vi "General Error Handler Core CORE__Copy.vi"(0 "[error code] (0)":i32 format="%0.0f", 1 "[error source] (\" \")":string, 3 "String to Format (not a refnum)":refnum<vi>, 4 "type of dialog (OK msg:1)":T2=enum."OK message", 5 "error in (no error)":errorcluster, 6 "[user-defined codes]":i32[](array[numeric]), 7 "[exception action] (none:0)":i32(ring) items=["no exception", "cancel error on match", "set error on match"], 8 "ni.com link visible (F)":bool, 9 "prompts":T1={"Error %d occurred at %s"="Error %d occurred at %s", "Warning %d occurred at %s"="Warning %d occurred at %s", "Possible reasons: %s"="<b>Possible reason(s):</b>\\n%s", "Error not listed"="This error code is undefined. Undefined errors might occur for a number of reasons. For example, no one has provided a description for the code, or you might have wired a number that is not an error code to the error code input. \n\nAdditionally, undefined error codes might occur because the error relates to a third-party object, such as the operating system or ActiveX. For these third-party errors, you might be able to obtain a description of the error by searching the Web for the error code (%s) or for its hexadecimal representation (0x%s).", "GetCommError x%lx"="Windows GetCommError:  The hex value of this code is <B>x%04lx</B>.\n\nInterpret it bit-wise as follows:\n<B>x4000</B>: serial port VI error\n<B>x0001</B>: receiving queue overflowed or character was received after end-of-file character\n<B>x0002</B>: character was lost by overwrite\n<B>x0004</B>: parity error\n<B>x0008</B>: framing error\n<B>x0010</B>: break condition\n<B>x0020</B>: CTS timeout\n<B>x0040</B>: DSR timeout\n<B>x0080</B>: RLSD timeout\n<B>x0100</B>: transmission queue was full when new character arrived\n<B>x0200</B>: parallel device timeout\n<B>x0400</B>: parallel device I/O error\n<B>x0800</B>: parallel device not selected\n<B>x1000</B>: parallel device out of paper\n<B>x8000</B>: requested mode is  not supported or the idComDev parameter is invalid.", "Continue"="Continue", "Stop"="Stop", "an unidentified location"="an unidentified location", "No Error"="No Error", "Help"="Why not found?"}, 10 "[user-defined descriptions]":string[](array[string]), 11 "[exception code]":i32 format="%0.0f", 13 "[exception source]":string) -> (12 "stop event propagated":bool, 14 "error?":bool, 15 "code out":i32 format="%0.0f", 17 "source out":string, 18 "message":string=" INSTRUCTIONS:\r\rNormal Use:  When using subVIs that incorporate the error in/error out (or error I/O) structure, place this handler where you want to inform the user of an error, typically at the end of the I/O data path, as the last action of the program.  If the error in error? is ERROR, the handler creates a message describing the error and its source.  If the type of dialog = 1 (default), the message is displayed to the user, who can only acknowledge it.  If the type = 2, the user can acknowledge the message or abort execution; aborting a program with active I/O is not recommended.  If the type = 0, no message is displayed; this is used to process the error programmatically, and the error out cluster elements are wired to individual terminals for that reason.  \r\rOther Use:\n\r\nlocal testing.  To test the error code of a subVI or function that does not have the error I/O structure, you can wire its error code and a source string to the local error code and error source inputs.  If error in error? indicates no error and error code is not equal to 0, the local code and source are substituted for the error in values, and error? is set TRUE (ERROR).", 19 "error out":errorcluster)   [LabVIEW 2020, in "Explain Error Improved Dialog.lvlib"]
uses:
  Explain Error Improved Dialog/Explain Error Improved Dialog.lvlib
  <vilib>/Utility/error.llb/DialogTypeEnum.ctl
  <vilib>/Utility/error.llb/whitespace.ctl
panel:
  # "reinitialize to default to display instructions"
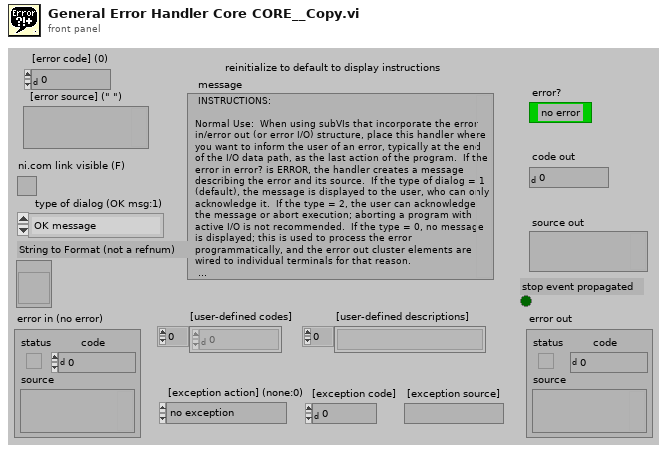
[diagram p1: front panel]
types:
  T1 = cluster{"Error %d occurred at %s":string, "Warning %d occurred at %s":string, "Possible reasons: %s":string, "Error not listed":string, "GetCommError x%lx":string, "Continue":string, "Stop":string, "an unidentified location":string, "No Error":string, "Help":string}
  T2 = typedef "DialogTypeEnum.ctl" = enum16{"no dialog", "OK message", "continue or stop message", "auto error handling dialog", "OK message + warnings", "continue/stop + warnings"}
  T3 = typedef "whitespace.ctl" = u16
  T4 = typedef "TagReturnType.ctl" = enum16{"No Tag", "<err>", "<append>"}
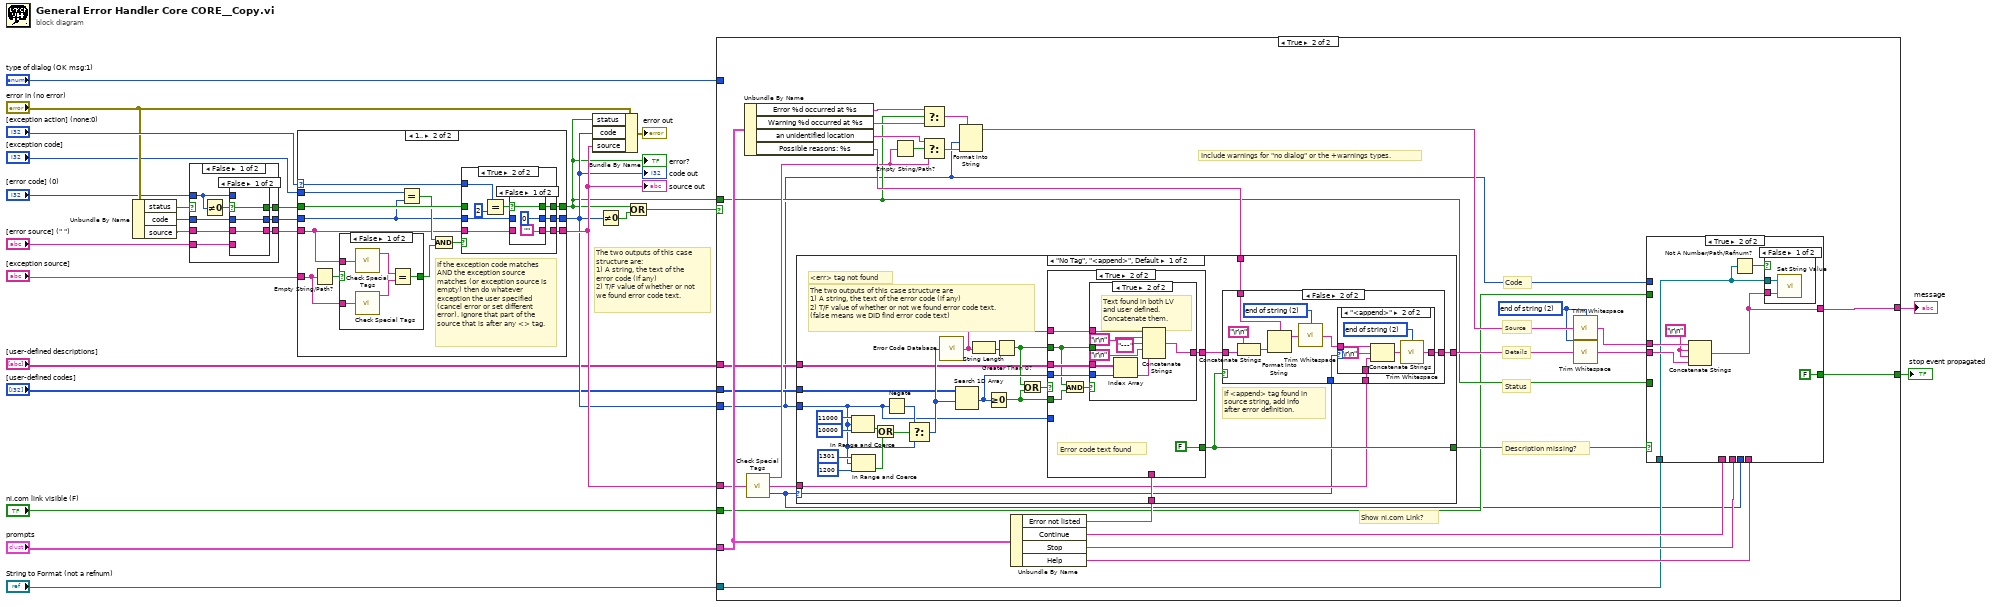
[diagram p0: block diagram]
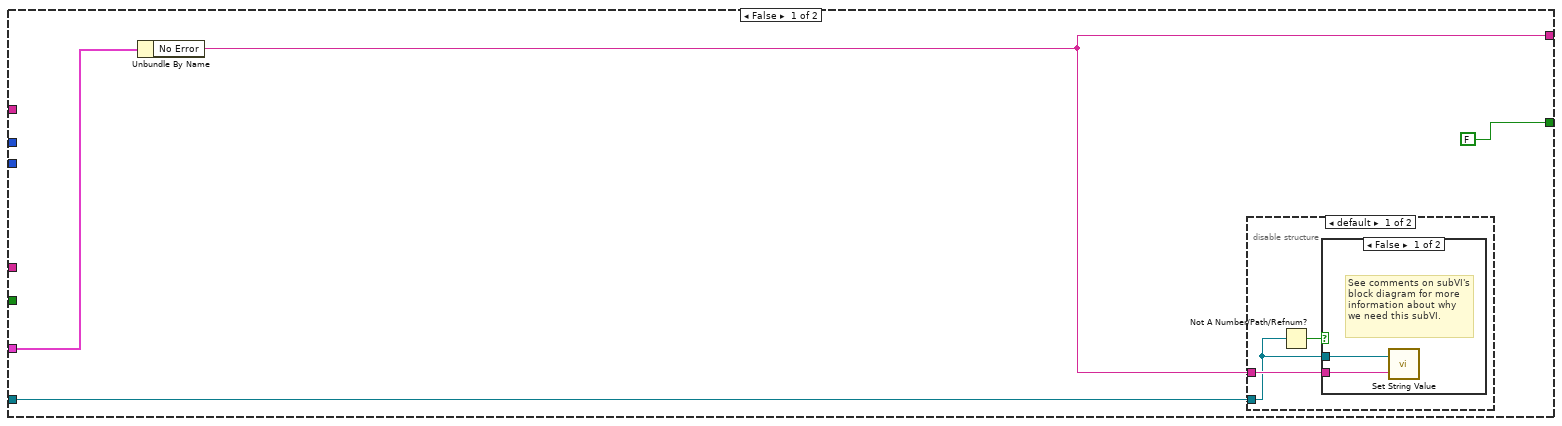
[diagram p8: hidden frame]
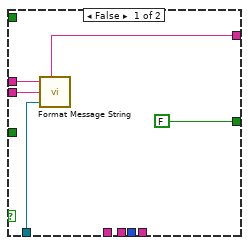
[diagram p11: hidden frame]
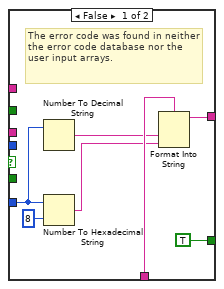
[diagram p15: hidden frame]
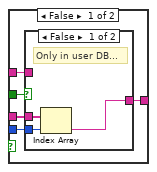
[diagram p16: hidden frame]
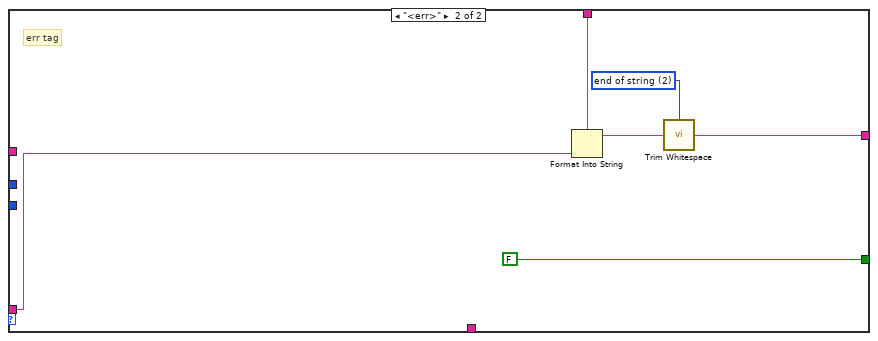
[diagram p18: hidden frame]
diagram:
  # "The two outputs of this case structure are:\n1) A string, the text of the error code (if any)\n2) T/F value of whether or not we found error code text."
  n1 = Unbundle By Name("error in (no error)") -> ("status"=w7:bool, "code"=w21:i32, "source"=w25:string)
  n2 = case shown="False" w7 {
    selector: w7 -> [_ w43]
    tunnel: [w32 w42] -> w23
    tunnel: [w33 w43] -> w22
    tunnel: w21 -> [w29 w42]
    tunnel: [w31 w41] -> w24
    tunnel: w25 -> [w30 w41]
    tunnel: "[error code] (0)" -> [w28 _]
    tunnel: "[error source] (\" \")" -> [w27 _]
    frame False {
      n3 = Not Equal To 0?(x=w28) -> (x != 0?=w34:bool)
      n4 = case shown="False" w34 {
        selector: w34 -> [w37 w40]
        tunnel: [w37 w40] -> w33
        tunnel: w28 -> [_ w39]
        tunnel: [w35 w39] -> w32
        tunnel: w27 -> [_ w38]
        tunnel: [w36 w38] -> w31
        tunnel: w30 -> [w36 _]
        tunnel: w29 -> [w35 _]
        frame False {
        }
        frame True {
        }
      }
    }
    frame True {
    }
  }
  n5 = case shown="1.." "[exception action] (none:0)" {
    selector: "[exception action] (none:0)" -> [_ w51]
    tunnel: [w46 w59] -> w3
    tunnel: w22 -> [w46 w57]
    tunnel: [w45 w58] -> w8
    tunnel: w23 -> [w45 w55]
    tunnel: [w44 w53] -> w18
    tunnel: w24 -> [w44 w49]
    tunnel: "[exception code]" -> [_ w52]
    tunnel: "[exception source]" -> [_ w48]
    frame ..0 {
    }
    frame 1.. {
      # "If the exception code matches AND the exception source matches (or exception source is empty) then do whatever exception the user specified (cancel error or set different error). Ignore that part of the source that is after any <> tag."
      n6 = Empty String/Path?(string/path=w48) -> (empty?=w50:bool)
      n7 = case shown="False" w50 {
        selector: w50 -> [_ w65]
        tunnel: w49 -> [w64 _]
        tunnel: w48 -> [w63 _]
        tunnel: [w62 w65] -> w47
        frame False {
          n8 = call <vilib>:"Check Special Tags.vi"("source"=w64) -> ("Before Tag (source)"=w61:string)  [unwired: 2 out]
          n9 = call <vilib>:"Check Special Tags.vi"("source"=w63) -> ("Before Tag (source)"=w60:string)  [unwired: 2 out]
          n10 = Equal?(x=w61, y=w60) -> (x = y?=w62:bool)
        }
        frame True {
          # "Empty string always matches."
        }
      }
      n11 = Equal?(x=w52, y=w55) -> (x = y?=w56:bool)
      n12 = And(x=w56, y=w47) -> (x .and. y?=w54:bool)
      n13 = case shown="True" w54 {
        tunnel: [w68 w69] -> w59
        tunnel: [w67 w73] -> w58
        tunnel: w57 -> [w68 _]
        tunnel: w55 -> [w67 w72]
        tunnel: w51 -> [_ w76]
        tunnel: [w66 w71] -> w53
        tunnel: w49 -> [w66 w70]
        frame False {
        }
        frame True {
          n14 = Equal?(x=w76, y=2) -> (x = y?=w74:bool)
          n15 = case shown="False" w74 {
            selector: w74 -> [w79 w82]
            tunnel: [0 w81] -> w73
            tunnel: w72 -> [_ w81]
            tunnel: ["" ("Empty String Constant") w80] -> w71
            tunnel: w70 -> [_ w80]
            tunnel: [w79 w82] -> w69
            frame False {
            }
            frame True {
            }
          }
        }
      }
    }
  }
  "source out" <- w18
  "error?" <- w3
  "code out" <- w8
  n16 = Bundle By Name(cluster="error in (no error)", "status"=w3, "code"=w8, "source"=w18) -> (→"error out":errorcluster)
  n17 = Not Equal To 0?(x=w8) -> (x != 0?=w2:bool)
  n18 = Or(x=w3, y=w2) -> (x .or. y?=w19:bool)
  n19 = case shown="True" w19 {
    tunnel: [w84 w107] -> w26
    tunnel: w3 -> [_ w98]
    tunnel: w18 -> [_ w103]
    tunnel: "prompts" -> [w86 w112]
    tunnel: [FALSE ("Stop 2") w109] -> w14
    tunnel: "String to Format (not a refnum)" -> [w83 w104]
    tunnel: w8 -> [_ w96]
    tunnel: "[user-defined descriptions]" -> [_ w100]
    tunnel: "[user-defined codes]" -> [_ w99]
    tunnel: "type of dialog (OK msg:1)" -> [_ _]
    tunnel: "ni.com link visible (F)" -> [_ w97]
    frame False {
      n20 = Unbundle By Name(w86) -> ("No Error"=w84:string)
      n21 = disable-structure shown="default" {
        disable-tunnel: w84 -> [w89 _]
        disable-tunnel: w83 -> [w88 _]
        frame condition #0 (active) {
          n22 = Not A Number/Path/Refnum?(number/path/refnum=w88) -> (NaN/Path/Refnum?=w87:bool)
          n23 = case shown="False" w87 {
            tunnel: w89 -> [w91 _]
            tunnel: w88 -> [w90 _]
            frame False {
              # "See comments on subVI's block diagram for more information about why we need this subVI."
              n24 = call <vilib>:"Set String Value.vi"("No Error"=w91, "String to Format (not a refnum)"=w90) -> ()
            }
            frame True {
            }
          }
        }
        frame condition #1 {
          # "Do nothing in RT case."
        }
      }
    }
    frame True {
      w92 = T3 2 items=["both", "start of string", "end of string"] ("location (both)")
      # "Code"
      # "Description missing?"
      # "Status"
      # "Details"
      # "Source"
      # "Show ni.com Link?"
      # "Include warnings for \"no dialog\" or the +warnings types."
      n25 = Unbundle By Name(w112) -> ("Error %d occurred at %s"=w101:string, "Warning %d occurred at %s"=w119:string, "an unidentified location"=w116:string, "Possible reasons: %s"=w108:string)
      n26 = call <vilib>:"Check Special Tags.vi"("source"=w103) -> ("Before Tag (source)"=w102:string, "After Tag (special data)"=w120:string, "Tag Found?"=w95:T4)
      n27 = Empty String/Path?(string/path=w102) -> (empty?=w121:bool)
      n28 = Select(t=w101, s=w98, f=w119) -> (s? t:f=w118:string)
      n29 = Select(t=w116, s=w121, f=w102) -> (s? t:f=w117:string)
      n30 = Format Into String(format string=w118, w96, w117) -> (resulting string=w105:string)  [unwired: 2 in, 1 out]
      n31 = Unbundle By Name(w112) -> ("Error not listed"=w115:string, "Continue"=w114:string, "Stop"=w113:string, "Help"=w110:string)
      n32 = case shown="\"No Tag\", \"<append>\", Default" w95 {
        selector: w95 -> [w136 _]
        tunnel: [w141 w214] -> w106
        tunnel: w96 -> [w137 _]
        tunnel: w120 -> [w142 w213]
        tunnel: w115 -> [w160 _]
        tunnel: [w143 FALSE] -> w111
        tunnel: w108 -> [w145 w212]
        tunnel: w100 -> [w139 _]
        tunnel: w99 -> [w138 _]
        frame "No Tag", "<append>", Default {
          # "If <append> tag found in source string, add info after error definition."
          # "<err> tag not found"
          # "The two outputs of this case structure are\n1) A string, the text of the error code (if any)\n2) T/F value of whether or not we found error code text.\n(false means we DID find error code text)"
          n33 = In Range and Coerce(upper limit=11000, x=w137, lower limit=10000) -> (In Range?=w153:bool)  [unwired: 1 out]
          n34 = In Range and Coerce(upper limit=1301, x=w137, lower limit=1200) -> (In Range?=w154:bool)  [unwired: 1 out]
          n35 = Or(x=w153, y=w154) -> (x .or. y?=w152:bool)
          n36 = Negate(x=w137) -> (-x=w156:i32)
          n37 = Select(t=w156, s=w152, f=w137) -> (s? t:f=w140:i32)
          n38 = call <vilib>:"Error Code Database.vi"("Error Code"=w140) -> ("Error Text"=w146:string)
          n39 = Search 1D Array(1D array=w138, element=w140) -> (index of element=w159:i32)  [unwired: 1 in]
          n40 = String Length(string=w146) -> (length=w150:i32)
          n41 = Greater Or Equal To 0?(x=w159) -> (x >= 0?=w147:bool)
          n42 = Greater Than 0?(x=w150) -> (x > 0?=w148:bool)
          n43 = Or(x=w148, y=w147) -> (x .or. y?=w149:bool)
          n44 = case shown="True" w149 {
            tunnel: w159 -> [_ w189]
            tunnel: [w183 w187] -> w144
            tunnel: w160 -> [w182 _]
            tunnel: [TRUE FALSE] -> w143
            tunnel: w148 -> [_ w186]
            tunnel: w147 -> [_ w191]
            tunnel: w139 -> [_ w190]
            tunnel: w146 -> [_ w188]
            tunnel: w137 -> [w179 _]
            frame False {
              # "The error code was found in neither the error code database nor the user input arrays."
              n45 = Number To Decimal String(number=w179) -> (decimal integer string=w180:string)  [unwired: 1 in]
              n46 = Number To Hexadecimal String(1:i16 8 ("width (-)"), 2:w179) -> (0:w181:string)
              n47 = Format Into String(format string=w182, w180, w181) -> (resulting string=w183:string)  [unwired: 2 in, 1 out]
            }
            frame True {
              # "Error code text found"
              n48 = And(x=w186, y=w191) -> (x .and. y?=w192:bool)
              n49 = case shown="True" w192 {
                tunnel: w190 -> [w195 w210]
                tunnel: w189 -> [w194 w209]
                tunnel: w188 -> [w196 w203]
                tunnel: [w197 w207] -> w187
                tunnel: w186 -> [w198 _]
                frame False {
                  n50 = case shown="False" w198 {
                    tunnel: [w199 w202] -> w197
                    tunnel: w196 -> [_ w202]
                    tunnel: w195 -> [w201 _]
                    tunnel: w194 -> [w200 _]
                    frame False {
                      # "Only in user DB..."
                      n51 = Index Array(array=w201, index=w200) -> (element=w199:string)
                    }
                    frame True {
                      # "Only in LV DB..."
                    }
                  }
                }
                frame True {
                  # "Text found in both LV\nand user defined. \nConcatenate them."
                  n52 = Index Array(array=w210, index=w209) -> (element=w208:string)
                  n53 = Concatenate Strings(w203, "\r\n" ("End of Line Constant"), "---" ("string"), "\r\n" ("End of Line Constant"), w208) -> (w207:string)
                }
              }
            }
          }
          n54 = case shown="False" w143 {
            tunnel: w145 -> [_ w171]
            tunnel: [w161 w163] -> w141
            tunnel: w144 -> [w161 w168]
            tunnel: w136 -> [_ w165]
            tunnel: w142 -> [_ w164]
            frame True {
              # "no explanation given for error."
            }
            frame False {
              w162 = T3 2 items=["both", "start of string", "end of string"] ("location (both)")
              n55 = Concatenate Strings("\r\n" ("End of Line Constant"), w168) -> (w169:string)
              n56 = Format Into String(format string=w171, w169) -> (resulting string=w170:string)  [unwired: 2 in, 1 out]
              n57 = call <vilib>:"Trim Whitespace.vi"("string"=w170, "location (both)"=w162) -> ("trimmed string"=w166:string)
              n58 = case shown="\"<append>\"" w165 {
                tunnel: w166 -> [w172 w177]
                tunnel: [w172 w174] -> w163
                tunnel: w164 -> [_ w176]
                frame "No Tag", Default {
                }
                frame "<append>" {
                  w173 = T3 2 items=["both", "start of string", "end of string"] ("location (both)")
                  n59 = Concatenate Strings(w177, "\r\n" ("End of Line Constant"), w176) -> (w175:string)
                  n60 = call <vilib>:"Trim Whitespace.vi"("string"=w175, "location (both)"=w173) -> ("trimmed string"=w174:string)
                }
              }
            }
          }
        }
        frame "<err>" {
          w211 = T3 2 items=["both", "start of string", "end of string"] ("location (both)")
          # "err tag"
          n61 = Format Into String(format string=w212, w213) -> (resulting string=w215:string)  [unwired: 2 in, 1 out]
          n62 = call <vilib>:"Trim Whitespace.vi"("string"=w215, "location (both)"=w211) -> ("trimmed string"=w214:string)
        }
      }
      n63 = call <vilib>:"Trim Whitespace.vi"("string"=w105, "location (both)"=w92) -> ("trimmed string"=w93:string)
      n64 = call <vilib>:"Trim Whitespace.vi"("string"=w106, "location (both)"=w92) -> ("trimmed string"=w94:string)
      n65 = case shown="True" w111 {
        tunnel: w94 -> [w125 w132]
        tunnel: w110 -> [_ _]
        tunnel: w114 -> [_ _]
        tunnel: w113 -> [_ _]
        tunnel: [FALSE ("stop event propagated") FALSE ("stop event propagated")] -> w109
        tunnel: w93 -> [w126 w133]
        tunnel: w98 -> [_ _]
        tunnel: [w122 w130] -> w107
        tunnel: w104 -> [w124 w128]
        tunnel: w97 -> [_ _]
        tunnel: w96 -> [_ _]
        tunnel: w95 -> [_ _]
        frame False {
          n66 = call <vilib>:"Format Message String.vi"("Source"=w126, "Details"=w125, "String to Format (not a refnum)"=w124) -> ("message"=w122:string)  [unwired: 1 in, 4 out]
        }
        frame True {
          w131 = "\r\n" ("End of Line Constant")
          n67 = Concatenate Strings(w133, w131, w131, w132) -> (w130:string)
          n68 = Not A Number/Path/Refnum?(number/path/refnum=w128) -> (NaN/Path/Refnum?=w129:bool)
          n69 = case shown="False" w129 {
            tunnel: w128 -> [w135 _]
            tunnel: w130 -> [w134 _]
            frame False {
              n70 = call <vilib>:"Set String Value.vi"("No Error"=w134, "String to Format (not a refnum)"=w135) -> ()
            }
            frame True {
            }
          }
        }
      }
    }
  }
  "message" <- w26
  "stop event propagated" <- w14
